vi "KERNEL32_error.vi"(7 "name":string, 9 "return":i32, 11 "error in (no error)":errorcluster) -> (3 "error out":errorcluster)   [LabVIEW 2020, in "JKI dotNET System Exec.lvlib" / "dotnet_system_exec.lvclass"]
uses:
  dotnet_system_exec.lvclass
  <vilib>/ErrorRing/Error Ring.xnode
  dotnet_system_exec.lvclass/dotnet_system_exec.ctl
  <vilib>/Utility/error.llb/Error Cluster From Error Code.vi
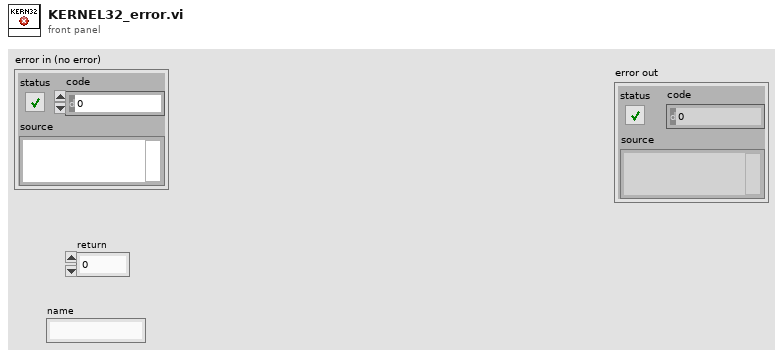
[diagram p1: front panel]
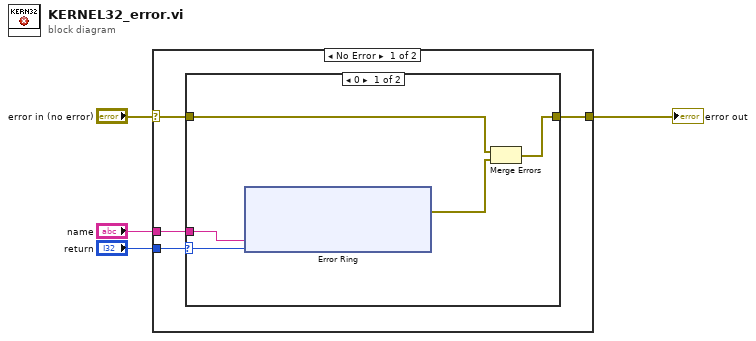
[diagram p0: block diagram]
diagram:
  n1 = case shown="No Error" "error in (no error)" {
    selector: "error in (no error)" -> [w7 w23]
    tunnel: [w6 w23] -> w3
    tunnel: "return" -> [w8 _]
    tunnel: "name" -> [w5 _]
    frame No Error {
      n2 = case shown="0" w8 {
        selector: w8 -> [w13 _]
        tunnel: w7 -> [w12 w22]
        tunnel: [w10 w22] -> w6
        tunnel: w5 -> [w9 _]
        frame 0 {
          n3 = xnode "Error Ring"("parameter 0"=w9, "parameter 1"=w13) -> ("error out"=w11:errorcluster)
          n4 = Merge Errors(w12, w11) -> (w10:errorcluster)
        }
        frame 1, Default {
        }
      }
    }
    frame Error {
    }
  }
  "error out" <- w3
